vi "OP500Z8P_MicroOCV.vi"(8 "errin":errorcluster) -> (0 "errout":errorcluster, 3 "OCV_PDU":dbl)   [LabVIEW 2020]
uses:
  <userlib>/PCAN Basic/Controls/BaudrateEenum.ctl
  <userlib>/PCAN Basic/Controls/Channel.ctl
  <userlib>/PCAN Basic/PCANBasic.lvlib
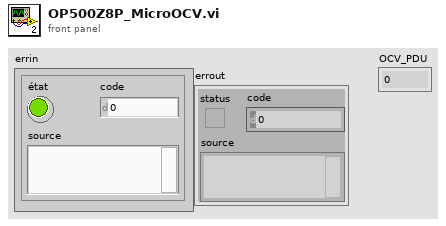
[diagram p1: front panel]
types:
  T1 = typedef "PCANBasic.lvlib/Channel.ctl" = enum16{"PCAN_NONEBUS", "not used1", "not used2", "not used3", "not used4", "not used5", "not used6", "not used7", "not used8", "not used9", "not used10", "not used11", "not used12", "not used13", "not used14", "not used15", "not used16", "not used17", "not used18", "not used19", "not used20", "not used21", "not used22", "not used23", "not used24", "not used25", "not used26", "not used27", "not used28", "not used29", "not used30", "not used31", "not used32", "PCAN_ISABUS1", "PCAN_ISABUS2", "PCAN_ISABUS3", "PCAN_ISABUS4", "PCAN_ISABUS5", "PCAN_ISABUS6", "PCAN_ISABUS7", "PCAN_ISABUS8", "not used41", "not used42", "not used43", "not used44", "not used45", "not used46", "not used47", "not used48", "PCAN_DNGBUS1", "not used50", "not used51", "not used52", "not used53", "not used54", "not used55", "not used56", "not used57", "not used58", "not used59", "not used60", "not used61", "not used62", "not used63", "not used64", "PCAN_PCIBUS1", "PCAN_PCIBUS2", "PCAN_PCIBUS3", "PCAN_PCIBUS4", "PCAN_PCIBUS5", "PCAN_PCIBUS6", "PCAN_PCIBUS7", "PCAN_PCIBUS8", "not used73", "not used74", "not used75", "not used76", "not used77", "not used78", "not used79", "not used80", "PCAN_USBBUS1", "PCAN_USBBUS2", "PCAN_USBBUS3", "PCAN_USBBUS4", "PCAN_USBBUS5", "PCAN_USBBUS6", "PCAN_USBBUS7", "PCAN_USBBUS8", "Not used89", "Not used90", "Not used91", "Not used92", "Not used93", "Not used94", "Not used95", "Not used96", "PCAN_PCCBUS1", "PCAN_PCCBUS2"}
  T2 = typedef "PCANBasic.lvlib/BaudrateEenum.ctl" = enum16{"CAN_Baud_1M", "CAN_Baud_800K", "CAN_BAUD_500K", "CAN_BAUD_250K", "CAN_BAUD_125K", "CAN_BAUD_100K", "CAN_BAUD_95K", "CAN_BAUD_83K", "CAN_BAUD_50K", "CAN_BAUD_47K", "CAN_BAUD_33K", "CAN_BAUD_20K", "CAN_BAUD_10K", "CAN_BAUD_5K", "User Baudrate"}
  T3 = typedef "PCANBasic.lvlib/CAN MSG Cluster.ctl" = cluster{"ID":u32, "MSG type":enum8{"STD", "RTR", "XTD", "XTD RTR", "STATUS"}, "LEN":i8, "DATA":u8[]}
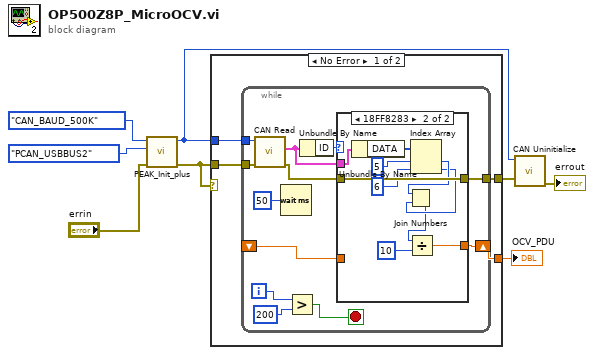
[diagram p0: block diagram]
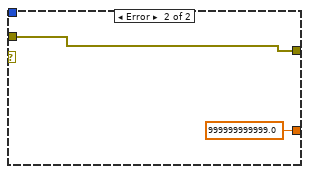
[diagram p3: hidden frame]
diagram:
  n1 = call <userlib>:"PEAK_Init_plus.vi"("errin"="errin", "Channel"=Channel."PCAN_USBBUS2", "BTR0BTR1"=BaudrateEenum."CAN_BAUD_500K") -> ("errout"=w3:errorcluster, "Channel out"=w2:T1)  [unwired: 7 in]
  n2 = case shown="No Error" w3 {
    tunnel: w3 -> [w12 w38]
    tunnel: [w11 w38] -> w5
    tunnel: w2 -> [w10 _]
    tunnel: [w9 999999999999.0] -> w1
    frame No Error {
      n3 = while {
        tunnel: w12 -> [w24]
        tunnel: w10 -> [w23]
        tunnel: [w19] -> w11
        shift-right: [w17] -> w9
        shift-left: _ -> [w16]
        i -> [w15]
        stop <- w13 stop-if-true
        n4 = call <userlib>:"CAN Read.vi"("error in (no error)"=w24, "Channel"=w23) -> ("error out"=w18:errorcluster, "CAN_Message out"=w21:T3)  [unwired: 5 in, 3 out]
        n5 = Wait (ms)(milliseconds to wait=u32 50) -> ()  [unwired: 1 out]
        n6 = Greater?(x=w15, y=200) -> (0:w13:bool)
        n7 = Unbundle By Name(w21) -> ("ID"=w22:u32)
        n8 = case shown="18FF8283" w22 {
          tunnel: w21 -> [_ w36]
          tunnel: [w26 w34] -> w19
          tunnel: w18 -> [w26 w34]
          tunnel: [w25 w27] -> w17
          tunnel: w16 -> [w25 _]
          frame 0, Default {
          }
          frame 419398275 {
            n9 = Unbundle By Name(w36) -> ("DATA"=w35:u8[])
            n10 = Index Array(array=w35, index #1=5 ("index"), index #2=6 ("index")) -> (element #1=w31:u8, element #2=w30:u8)
            n11 = Join Numbers(hi=w31, lo=w30) -> ((hi.lo)=w29:u16)
            n12 = Divide(x=w29, y=u16 10) -> (x/y=w27:dbl)
          }
        }
      }
    }
    frame Error {
    }
  }
  "OCV_PDU" <- w1
  n13 = call <userlib>:"CAN Uninitialize.vi"("error in (no error)"=w5, "Channel"=w2) -> ("error out"=→"errout":errorcluster)  [unwired: 7 in, 2 out]
